vi "FitGaussian (SubVI).vi"(0 "Normalized Intensity vs Radius in":cluster{dbl[], dbl[]}, 1 "x values":dbl[](array[numeric]), 2 "y values":dbl[](array[numeric]), 3 "Estimated mean":dbl, 4 "Estimated width":dbl, 6 "initial guess":T1={"initial amplitude"=nan, "initial center"=nan, "initial standard deviation"=nan, "offset"=nan}, 7 "Nsigma Low":dbl=4.0 format="%#_13g", 8 "Use all points":bool, 9 "Nsigma High":dbl=4.0 format="%#_13g") -> (14 "data plot":cluster{dbl[], dbl[]}(graph), 15 "derivative data plot with Gaussian fit":T2(graph), 16 "amplitude":dbl, 17 "center":dbl, 18 "standard deviation":dbl, 19 "residue":dbl)   [LabVIEW 2016]
uses:
  <vilib>/Analysis/NI_AALPro.lvlib
panel:
  # "RESULTS"
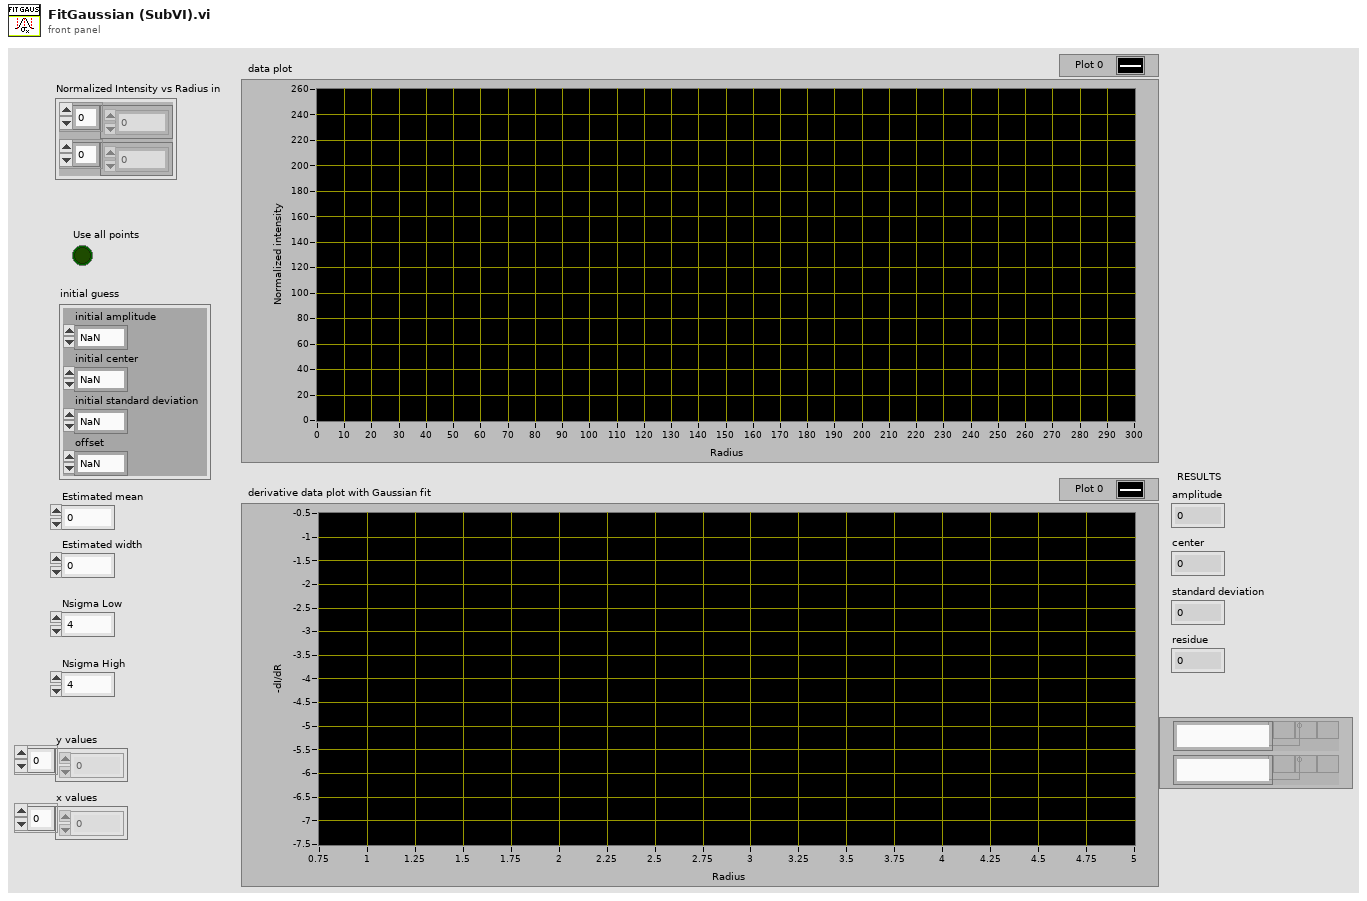
[diagram p1: front panel]
types:
  T1 = cluster{"initial amplitude":dbl, "initial center":dbl, "initial standard deviation":dbl, "offset":dbl}
  T2 = cluster{"Radius bins":dbl[], "Best Gaussian Fit":dbl[]}[]
  T3 = cluster{"x values":dbl[], "Best Gaussian Fit":dbl[]}
  T4 = cluster{"x values":dbl[], "Best Gaussian Fit":dbl[]}[]
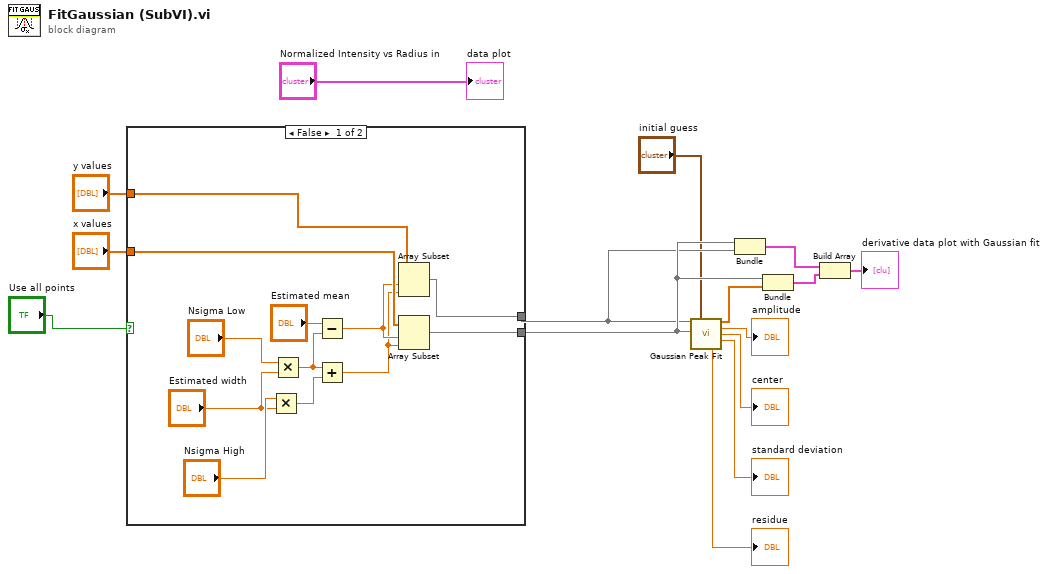
[diagram p0: block diagram]
diagram:
  n1 = case shown="False" "Use all points" {
    tunnel: "y values" -> [w25 w28]
    tunnel: [w24 w28] -> w3
    tunnel: "x values" -> [w23 w29]
    tunnel: [w22 w29] -> w6
    frame False {
      n2 = Multiply(x="Nsigma High", y="Estimated width") -> (x*y=w17:dbl)
      n3 = Multiply(x="Nsigma Low", y="Estimated width") -> (x*y=w18:dbl)
      n4 = Subtract(x="Estimated mean", y=w18) -> (x-y=w21:dbl)
      n5 = Add(x=w18, y=w17) -> (x+y=w16:dbl)
      n6 = Array Subset(array=w25, index=w21, length=w16) -> (w24:dbl[])
      n7 = Array Subset(array=w23, index=w21, length=w16) -> (w22:dbl[])
    }
    frame True {
    }
  }
  n8 = call <vilib>:"Gaussian Peak Fit.vi"("Y"=w3, "initial guess"="initial guess", "X"=w6) -> ("Best Gaussian Fit"=w14:dbl[], "amplitude"=→"amplitude":dbl, "center"=→"center":dbl, "standard deviation"=→"standard deviation":dbl, "residue"=→"residue":dbl)  [unwired: 6 in, 2 out]
  n9 = Bundle("x values"=w6, "y values"=w3) -> (w4:cluster{"x values":dbl[], "y values":dbl[]})  [unwired: 1 in]
  n10 = Bundle("x values"=w6, "Best Gaussian Fit"=w14) -> (w13:T3)  [unwired: 1 in]
  n11 = Build Array(w4, w13) -> (→"derivative data plot with Gaussian fit":T4)
  "data plot" <- "Normalized Intensity vs Radius in"
